vi "SPTSequenceBulilder.vi"(10 "Number Of Operations":i32, 11 "Proocessing Times MxJ":u16[][](array[numeric])) -> (2 "SPT Sequence":i32[](array[numeric]), 3 "Flattened Processing Times":u16[](array[numeric]))   [LabVIEW 2013]
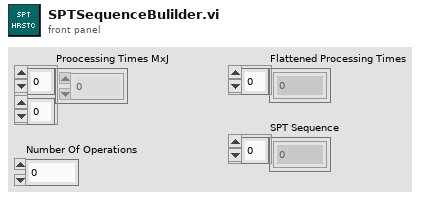
[diagram p1: front panel]
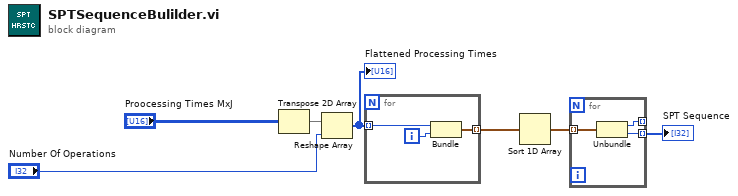
[diagram p0: block diagram]
diagram:
  n1 = Transpose 2D Array(2D array="Proocessing Times MxJ") -> (transposed array=w2:u16[][])
  n2 = Reshape Array(w2, "Number Of Operations") -> (w5:u16[])
  "Flattened Processing Times" <- w5
  n3 = for {
    tunnel: w5 -> [w10] mode=indexing
    tunnel: [w8] -> w3 mode=indexing
    i -> [w9]
    n4 = Bundle(w10, w9) -> (w8:cluster{u16, i32})  [unwired: 1 in]
  }
  n5 = Sort 1D Array(array=w3) -> (sorted array=w1:cluster{u16, i32}[])
  n6 = for {
    tunnel: w1 -> [w13] mode=indexing
    tunnel: [w12] -> _ mode=indexing
    tunnel: [w11] -> w6 mode=indexing
    n7 = Unbundle(w13) -> (w12:u16, w11:i32)
  }
  "SPT Sequence" <- w6
